vi "KeysightMeasCurr.vi"(8 "error in (no error)":errorcluster, 11 "VISA resource name":refnum<visa-resource-name>) -> (0 "error out":errorcluster, 2 "CURR":dbl, 3 "VISA resource name out":refnum<visa-resource-name>)   [LabVIEW 2017]
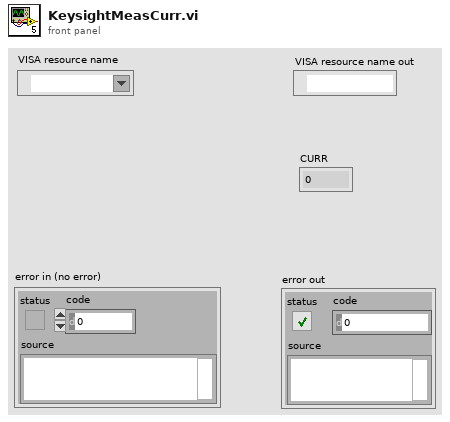
[diagram p1: front panel]
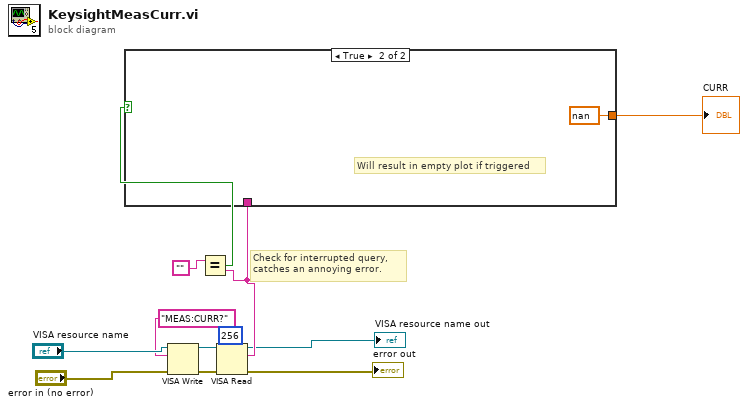
[diagram p0: block diagram]
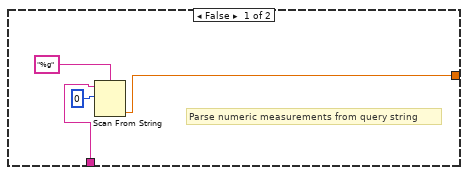
[diagram p2: hidden frame]
diagram:
  # "Check for interrupted query, \ncatches an annoying error."
  n1 = VISA Write(VISA resource name="VISA resource name", write buffer="MEAS:CURR?", error in (no error)="error in (no error)") -> (VISA resource name out=w9:refnum<visa-resource-name>, error out=w8:errorcluster)  [unwired: 1 out]
  n2 = VISA Read(VISA resource name=w9, byte count=u32 256, error in (no error)=w8) -> (VISA resource name out=→"VISA resource name out":refnum<visa-resource-name>, read buffer=w4:string, error out=→"error out":errorcluster)  [unwired: 1 out]
  n3 = Equal?(x="", y=w4) -> (x = y?=w5:bool)
  n4 = case shown="True" w5 {
    tunnel: w4 -> [w14 _]
    tunnel: [w13 nan] -> w1
    frame False {
      # "Parse numeric measurements from query string"
      n5 = Scan From String(format string="%g", input string=w14, initial scan location=u32 0) -> (output 1=w13:dbl)  [unwired: 2 in, 3 out]
    }
    frame True {
      # "Will result in empty plot if triggered"
    }
  }
  "CURR" <- w1
